vi "WILT SS Current Test.vi"(6 "Lower Limit 2":dbl[](array[numeric])=[18.0, 18.0, 18.0, 18.0, 18.0, 18.0, 18.0, 18.0, 18.0, -1.0, -1.0, -1.0, -1.0, -1.0, -1.0, -1.0, -1.0, -1.0, 3.6, 3.6, 3.6, 3.6, 3.6, 3.6, -1.0, -1.0, -1.0, -1.0], 8 "Lower Limit":dbl[](array[numeric])=[18.0, 18.0, 18.0, 18.0, 18.0, 18.0, 18.0, 18.0, 18.0, -1.0, -1.0, -1.0, -1.0, -1.0, -1.0, -1.0, -1.0, -1.0, 3.6, 3.6, 3.6, 3.6, 3.6, 3.6, -1.0, -1.0, -1.0, -1.0], 9 "Y 2":dbl[](array[numeric]), 10 "Y":dbl[](array[numeric]), 11 "Upper Limit":dbl[](array[numeric])=[50.0, 50.0, 27.0, 27.0, 27.0, 27.0, 27.0, 27.0, 27.0, 27.0, 27.0, 1.0, 1.0, 1.0, 1.0, 1.0, 4.4, 4.4, 4.4, 4.4, 4.4, 4.4, 4.4, 4.4, 4.4, 4.4, 1.0, 1.0]) -> (2 "Out of Bounds":bool, 3 "Waveform Chart":waveform(dbl)[](graph))   [LabVIEW 2016]
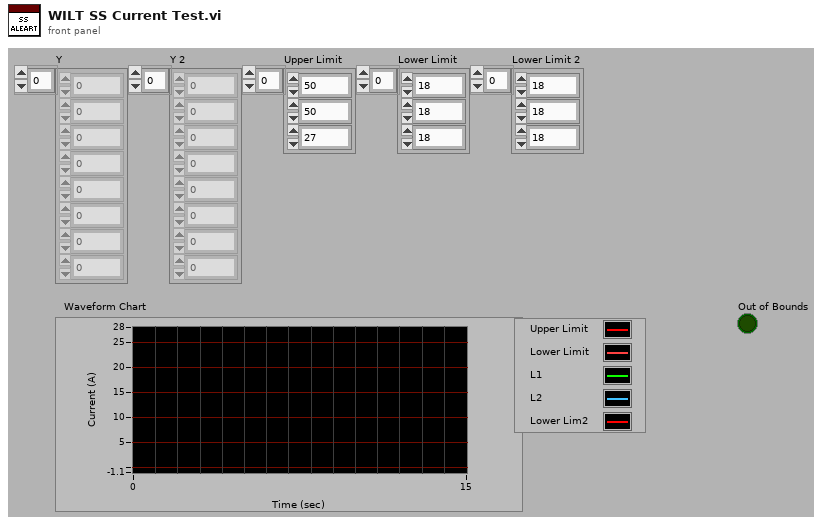
[diagram p1: front panel]
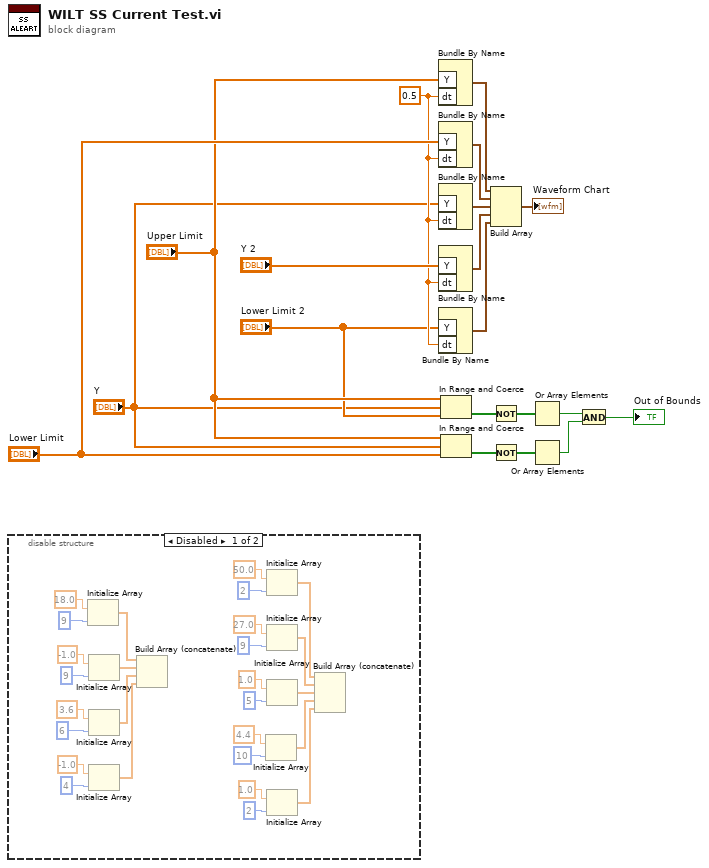
[diagram p0: block diagram]
diagram:
  w10 = 0.5 ("dt")
  n1 = disable-structure shown="Disabled" {
    frame Disabled {
      n2 = Initialize Array(18.0, 9 ("dimension size")) -> (w35:dbl[])
      n3 = Initialize Array(-1.0, 9 ("dimension size")) -> (w36:dbl[])
      n4 = Initialize Array(3.6 ("y"), 6 ("dimension size")) -> (w37:dbl[])
      n5 = Initialize Array(-1.0, 4 ("dimension size")) -> (w38:dbl[])
      n6 = Build Array (concatenate)(w35, w36, w37, w38) -> ()  [unwired: 1 out]
      n7 = Initialize Array(4.4, 10 ("dimension size")) -> (w28:dbl[])
      n8 = Initialize Array(50.0, 2 ("dimension size")) -> (w31:dbl[])
      n9 = Initialize Array(27.0, 9 ("dimension size")) -> (w30:dbl[])
      n10 = Initialize Array(1.0 ("y"), 5 ("dimension size")) -> (w29:dbl[])
      n11 = Initialize Array(1.0 ("y"), 2 ("dimension size")) -> (w34:dbl[])
      n12 = Build Array (concatenate)(w31, w30, w29, w28, w34) -> ()  [unwired: 1 out]
    }
    frame Enabled {
    }
  }
  n13 = Bundle By Name("Y"="Upper Limit", "dt"=w10) -> (w19:waveform(dbl))  [unwired: 1 in]
  n14 = Bundle By Name("Y"="Lower Limit", "dt"=w10) -> (w17:waveform(dbl))  [unwired: 1 in]
  n15 = Bundle By Name("Y"="Y", "dt"=w10) -> (w16:waveform(dbl))  [unwired: 1 in]
  n16 = Bundle By Name("Y"="Y 2", "dt"=w10) -> (w11:waveform(dbl))  [unwired: 1 in]
  n17 = Bundle By Name("Y"="Lower Limit 2", "dt"=w10) -> (w9:waveform(dbl))  [unwired: 1 in]
  n18 = In Range and Coerce(upper limit="Upper Limit", x="Y", lower limit="Lower Limit 2") -> (In Range?=w5:bool[])  [unwired: 1 out]
  n19 = In Range and Coerce(upper limit="Upper Limit", x="Y", lower limit="Lower Limit") -> (In Range?=w14:bool[])  [unwired: 1 out]
  n20 = Build Array(w19, w17, w16, w11, w9) -> (→"Waveform Chart":waveform(dbl)[])
  n21 = Not(x=w5) -> (.not. x?=w4:bool[])
  n22 = Not(x=w14) -> (.not. x?=w13:bool[])
  n23 = Or Array Elements(Boolean array=w4) -> (logical OR=w1:bool)
  n24 = Or Array Elements(Boolean array=w13) -> (logical OR=w2:bool)
  n25 = And(x=w1, y=w2) -> (x .and. y?=→"Out of Bounds":bool)
